vi "command_as_admin.vi"(8 "error in (no error)":errorcluster, 10 "arguments":string, 11 "command":path) -> (0 "error out":errorcluster)   [LabVIEW 2015, in "lv-bin-windows.lvlib" / "v1.lvlib"]
uses:
  v1.lvlib
  <userlib>/antonio-alexander/lv-bin/lv-bin/public/api/v1/v1.lvlib
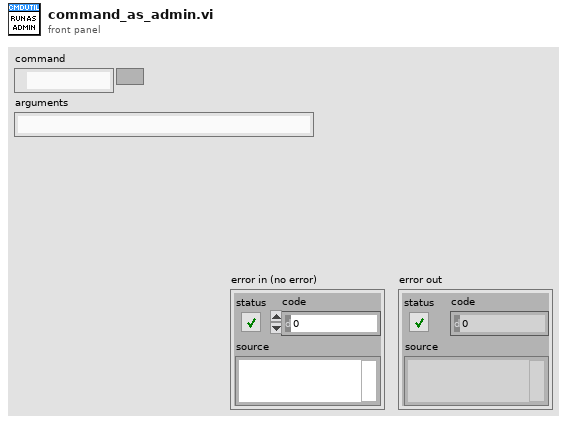
[diagram p1: front panel]
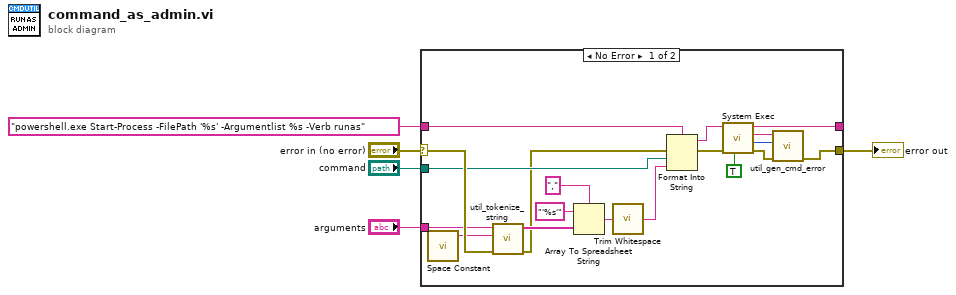
[diagram p0: block diagram]
diagram:
  n1 = case shown="No Error" "error in (no error)" {
    selector: "error in (no error)" -> [w19 w25]
    tunnel: "powershell.exe Start-Process -FilePath '%s' -Argumentlist %s -Verb runas" ("format string") -> [w18 _]
    tunnel: [w24 w25] -> w4
    tunnel: [w23 _] -> _
    tunnel: "command" -> [w13 _]
    tunnel: "arguments" -> [w17 _]
    frame No Error {
      n2 = call <vilib>:"Space Constant.vi"() -> ("String"=w10:string)
      n3 = call <userlib>:"util_tokenize_string.vi"("error in (no error)"=w19, "delimiter"=w10, "input_string"=w17) -> ("error out"=w12:errorcluster, "before_match []"=w16:string[])  [unwired: 6 in, 1 out]
      n4 = Array To Spreadsheet String(delimiter (Tab)=",", array=w16, 3:"'%s'" ("format string")) -> (spreadsheet string=w9:string)
      n5 = call <vilib>:"Trim Whitespace.vi"("string"=w9) -> ("trimmed string"=w8:string)  [unwired: 1 in]
      n6 = Format Into String(format string=w18, error in=w12, w13, w8) -> (resulting string=w22:string, error out=w11:errorcluster)  [unwired: 1 in]
      n7 = call <vilib>:"System Exec.vi"("run minimized? (F)"=TRUE, "error in (no error)"=w11, "command line"=w22) -> ("error out"=w20:errorcluster, "return code"=w6:i32, "standard error"=w7:string, "standard output"=w23:string)  [unwired: 5 in]
      n8 = call <userlib>:"util_gen_cmd_error.vi"("error in (no error)"=w20, "return_code"=w6, "standard_error"=w7) -> ("error out"=w24:errorcluster)  [unwired: 8 in]
    }
    frame Error {
    }
  }
  "error out" <- w4
